vi "FGV.vi"(6 "FGV state":T3, 8 "error in":errorcluster caption="entrée d'erreur") -> (0 "error out":errorcluster caption="sortie d'erreur", 3 "Local":T1)   [LabVIEW 2020]
doc: "FGV du projet"
uses:
  Ctrl/Ctrl_FGV_state.ctl
  Ctrl/Ctrl_FGV_Local.ctl
  Ctrl/Ctrl_data_ini.ctl
  Ctrl/Ctrl_INI_state.ctl
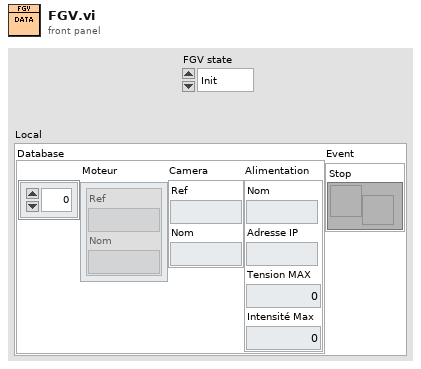
[diagram p1: front panel]
types:
  T1 = typedef "Ctrl_FGV_Local.ctl" = cluster{"Database":T2, "Event":cluster{"Stop ":refnum<user-event>}}
  T2 = typedef "Ctrl_data_ini.ctl" = cluster{"Moteur":cluster{"Ref":string, "Nom":string}[], "Camera":cluster{"Ref":string, "Nom":string}, "Alimentation":cluster{"Nom ":string, "Adresse IP ":string, "Tension MAX":u8, "Intensité Max":dbl}}
  T3 = typedef "Ctrl_FGV_state.ctl" = enum16{"Init", "Read", "Write File", "Read File"}
  T4 = typedef "Ctrl_INI_state.ctl" = enum16{"Read", "Write"}
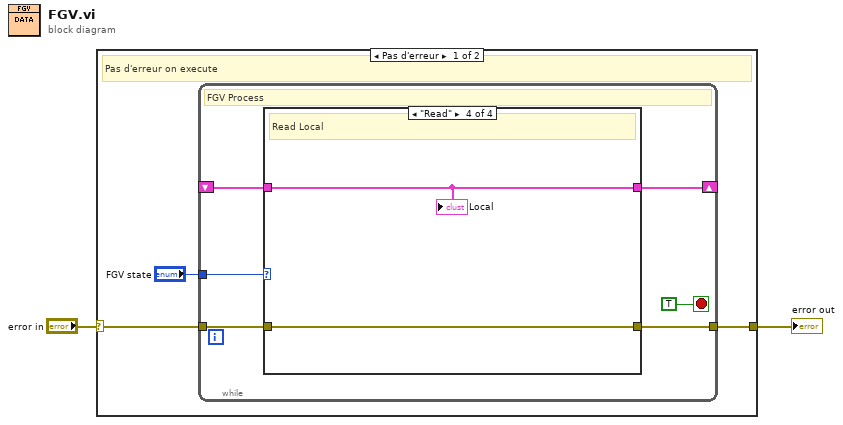
[diagram p0: block diagram]
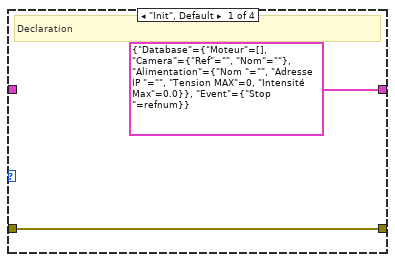
[diagram p2: hidden frame]
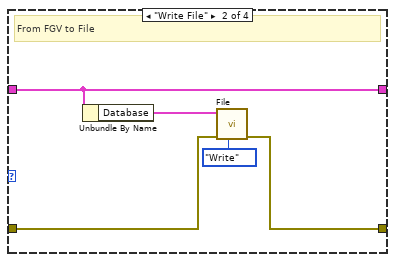
[diagram p3: hidden frame]
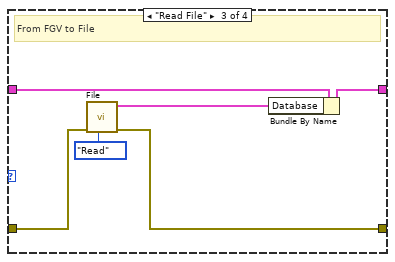
[diagram p4: hidden frame]
diagram:
  n1 = case shown="Pas d'erreur" "error in" {
    selector: "error in" -> [w5 w27]
    tunnel: [w4 w27] -> w1
    frame No Error {
      # "Pas d'erreur on execute"
      n2 = while {
        shift-right: [w7] -> _
        shift-left: _ -> [w6]
        tunnel: w5 -> [w10]
        tunnel: [w9] -> w4
        tunnel: "FGV state" -> [w8]
        stop <- TRUE stop-if-true
        # "FGV Process"
        n3 = case shown="\"Read\"" w8 {
          tunnel: w10 -> [w13 w17 w23 w26]
          tunnel: [w13 w16 w22 w26] -> w9
          tunnel: [T1 {"Database"={"Moteur"=[], "Camera"={"Ref"="", "Nom"=""}, "Alimentation"={"Nom "="", "Adresse IP "="", "Tension MAX"=0, "Intensité Max"=0.0}}, "Event"={"Stop "=refnum}} ("Local") w15 w20 w25] -> w7
          tunnel: w6 -> [_ w15 w21 w25]
          frame "Init", Default {
            # "Declaration"
          }
          frame "Write File" {
            # "From FGV to File"
            n4 = Unbundle By Name(w15) -> ("Database"=w14:T2)
            n5 = call "File.vi"("Ini_State"=Ctrl_INI_state."Write", "error in"=w17, "Valeur Write"=w14) -> ("error out"=w16:errorcluster)  [unwired: 7 in, 1 out]
          }
          frame "Read File" {
            # "From FGV to File"
            n6 = call "File.vi"("Ini_State"=Ctrl_INI_state."Read", "error in"=w23) -> ("error out"=w22:errorcluster, "Valeur Read"=w19:T2)  [unwired: 8 in]
            n7 = Bundle By Name(cluster=w21, "Database"=w19) -> (w20:T1)
          }
          frame "Read" {
            # "Read Local"
            "Local" <- w25
          }
        }
      }
    }
    frame Error {
      # "Erreur on laisse passer"
    }
  }
  "error out" <- w1
